vi "SRV_PM_App Initialization Routine.vi"(6 "Packet Mode Enable (T)":bool=TRUE, 7 "Read Response (F)":bool, 8 "error in (no error)":errorcluster, 9 "timeout ms (25,000)":i32=25000, 11 "connection ID":refnum<k5>) -> (0 "error out":errorcluster, 1 "Command Sent":string, 3 "connection ID out":refnum<k5>, 5 "Response":string)   [LabVIEW 2014]
uses:
  TCP_Communication/SRV_TCP Settings.ctl
  TCP_Communication/SRV_Package Methods.ctl
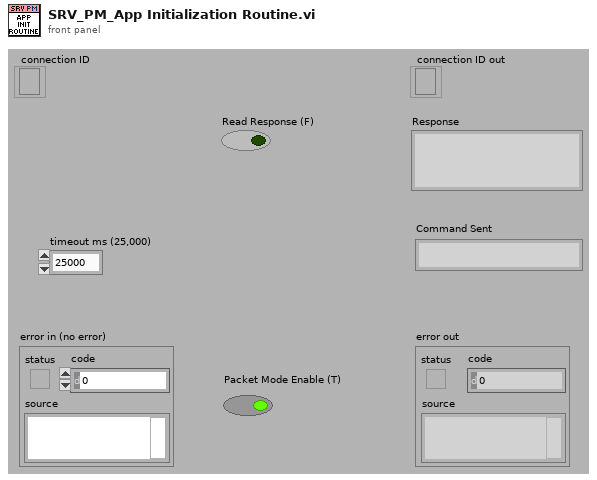
[diagram p1: front panel]
types:
  T1 = typedef "SRV_TCP Settings.ctl" = cluster{"Method":T2, "bytes to read":i32, "timeout ms (1000)":i32}
  T2 = typedef "SRV_Package Methods.ctl" = enum16{"General", "Standard", "CRLF", "Image", "HTML"}
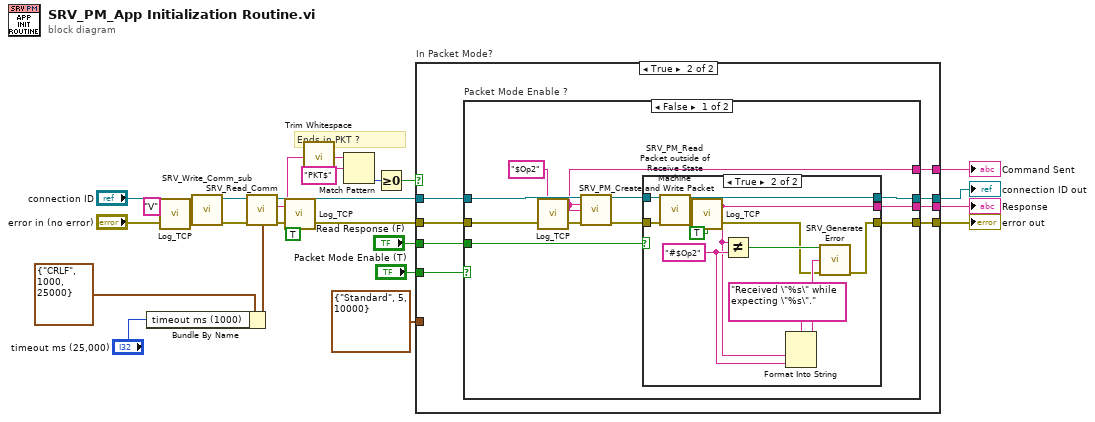
[diagram p0: block diagram]
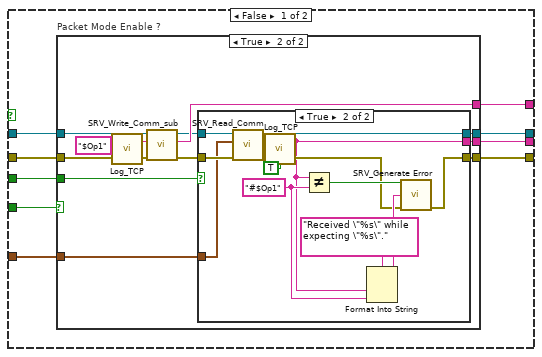
[diagram p2: hidden frame]
diagram:
  # "Ends in PKT ?"
  n1 = Bundle By Name(cluster=T1 {"Method"=enum."CRLF", "bytes to read"=1000, "timeout ms (1000)"=25000} ("TCP Settings"), "timeout ms (1000)"="timeout ms (25,000)") -> (w2:T1)
  n2 = call "Log_TCP.vi"("Data"="V" ("Command Sent"), "error in (no error)"="error in (no error)") -> ("Data dup"=w8:string, "error out"=w10:errorcluster)  [unwired: 12 in]
  n3 = call "SRV_Write_Comm_sub.vi"("error in (no error)"=w10, "Command Sent"=w8, "SRV In"="connection ID") -> ("error out"=w12:errorcluster, "SRV Out"=w25:refnum<k5>)  [unwired: 6 in, 1 out]
  n4 = call "SRV_Read_Comm.vi"("error in (no error)"=w12, "TCP Settings"=w2, "SRV In"=w25) -> ("error out"=w7:errorcluster, "Data out"=w5:string, "SRV Out"=w19:refnum<k5>)  [unwired: 6 in]
  n5 = call "Log_TCP.vi"("Data"=w5, "error in (no error)"=w7, "Response? (F: LV Writes)"=TRUE) -> ("error out"=w6:errorcluster)  [unwired: 11 in, 1 out]
  n6 = call <vilib>:"Trim Whitespace.vi"("string"=w5) -> ("trimmed string"=w24:string)  [unwired: 1 in]
  n7 = Match Pattern(string=w24, regular expression="PKT$") -> (offset past match=w22:i32)  [unwired: 1 in, 3 out]
  n8 = Greater Or Equal To 0?(x=w22) -> (x >= 0?=w21:bool)
  n9 = case "In Packet Mode?" shown="True" w21 {
    tunnel: w6 -> [w35 w73]
    tunnel: "Packet Mode Enable (T)" -> [w31 w74]
    tunnel: [w34 w72] -> w18
    tunnel: w19 -> [w32 w71]
    tunnel: [w33 w70] -> w17
    tunnel: [w30 w69] -> w16
    tunnel: "Read Response (F)" -> [w27 w68]
    tunnel: [w29 w67] -> w14
    tunnel: T1 {"Method"=enum."Standard", "bytes to read"=5, "timeout ms (1000)"=10000} ("TCP Settings") -> [w28 _]
    frame False {
      n10 = case "Packet Mode Enable ?" shown="True" w31 {
        tunnel: w35 -> [w36 w41]
        tunnel: [w36 w46] -> w34
        tunnel: w32 -> [w37 w50]
        tunnel: [w37 w47] -> w33
        tunnel: [_ w49] -> w30
        tunnel: [_ w48] -> w29
        tunnel: w28 -> [_ w43]
        tunnel: w27 -> [_ w42]
        frame False {
        }
        frame True {
          n11 = call "Log_TCP.vi"("Data"="$Op1", "error in (no error)"=w41) -> ("Data dup"=w38:string, "error out"=w40:errorcluster)  [unwired: 12 in]
          n12 = call "SRV_Write_Comm_sub.vi"("error in (no error)"=w40, "Command Sent"=w38, "SRV In"=w50) -> ("error out"=w45:errorcluster, "Command Sent dup"=w49:string, "SRV Out"=w44:refnum<k5>)  [unwired: 6 in]
          n13 = case shown="True" w42 {
            tunnel: w45 -> [w51 w66]
            tunnel: [w51 w58] -> w46
            tunnel: w44 -> [w52 w65]
            tunnel: [w52 w64] -> w47
            tunnel: w43 -> [_ w63]
            tunnel: [_ w54] -> w48
            frame False {
            }
            frame True {
              w60 = "#$Op1" ("y")
              n14 = call "SRV_Read_Comm.vi"("error in (no error)"=w66, "TCP Settings"=w63, "SRV In"=w65) -> ("error out"=w57:errorcluster, "Data out"=w55:string, "SRV Out"=w64:refnum<k5>)  [unwired: 6 in]
              n15 = call "Log_TCP.vi"("Data"=w55, "error in (no error)"=w57, "Response? (F: LV Writes)"=TRUE) -> ("Data dup"=w54:string, "error out"=w56:errorcluster)  [unwired: 11 in]
              n16 = Not Equal?(x=w54, y=w60) -> (x != y?=w62:bool)
              n17 = Format Into String(format string="Received \"%s\" while expecting \"%s\".", w54, w60) -> (resulting string=w59:string)  [unwired: 2 in, 1 out]
              n18 = call "SRV_Generate Error.vi"("status (T)"=w62, "Message"=w59, "error in (no error)"=w56) -> ("error out"=w58:errorcluster)  [unwired: 12 in]
            }
          }
        }
      }
    }
    frame True {
      n19 = case "Packet Mode Enable ?" shown="False" w74 {
        tunnel: w73 -> [w77 w102]
        tunnel: [w83 w102] -> w72
        tunnel: w71 -> [w85 w101]
        tunnel: [w81 w101] -> w70
        tunnel: [w75 _] -> w69
        tunnel: w68 -> [w80 _]
        tunnel: [w79 _] -> w67
        frame False {
          n20 = call "Log_TCP.vi"("Data"="$Op2", "error in (no error)"=w77) -> ("Data dup"=w75:string, "error out"=w78:errorcluster)  [unwired: 12 in]
          n21 = call "SRV_PM_Create and Write Packet.vi"("SRV ref"=w85, "Command Type"=w75, "Data String"=w75, "error in (no error)"=w78) -> ("SRV ref out"=w82:refnum<k5>, "error out"=w84:errorcluster)  [unwired: 10 in]
          n22 = case shown="True" w80 {
            tunnel: w84 -> [w86 w95]
            tunnel: [w86 w100] -> w83
            tunnel: w82 -> [w87 w94]
            tunnel: [w87 w93] -> w81
            tunnel: [_ w89] -> w79
            frame False {
            }
            frame True {
              w97 = "#$Op2" ("y")
              n23 = call "SRV_PM_Read Packet outside of Receive State Machine.vi"("SRV"=w94, "error in (no error)"=w95) -> ("SRV out"=w93:refnum<k5>, "Packet Data Field String"=w90:string, "error out"=w92:errorcluster)  [unwired: 9 in, 2 out]
              n24 = call "Log_TCP.vi"("Data"=w90, "error in (no error)"=w92, "Response? (F: LV Writes)"=TRUE) -> ("Data dup"=w89:string, "error out"=w91:errorcluster)  [unwired: 11 in]
              n25 = Not Equal?(x=w89, y=w97) -> (x != y?=w99:bool)
              n26 = Format Into String(format string="Received \"%s\" while expecting \"%s\".", w89, w97) -> (resulting string=w96:string)  [unwired: 2 in, 1 out]
              n27 = call "SRV_Generate Error.vi"("status (T)"=w99, "Message"=w96, "error in (no error)"=w91) -> ("error out"=w100:errorcluster)  [unwired: 12 in]
            }
          }
        }
        frame True {
        }
      }
    }
  }
  "connection ID out" <- w17
  "error out" <- w18
  "Command Sent" <- w16
  "Response" <- w14
